vi "Main.vi"() -> ()   [LabVIEW 2014]
uses:
  SubVI/Configs/Temp/TempConfig.ctl
  SubVI/Configs/Count/Channel.ctl
  <vilib>/Utility/miscctls.llb/LVForegroundBackgroundColorsTypeDef.ctl
  SubVI/VBreakInitialCond.ctl
  SubVI/VBreakStopCondition.ctl
  <instrlib>/Agilent 532XX Series/Public/Configure/Measurement/Configure Measurement (Totalize Timed).vi
  <instrlib>/Agilent 532XX Series/Public/Configure/Configure Channel (Slop).vi
  <instrlib>/Agilent 532XX Series/Public/Configure/Configure Channel (Auto Threshold Voltage).vi
  <instrlib>/Agilent 532XX Series/Public/Data/Read Measurement (Statistics).vi
  <instrlib>/Agilent 532XX Series/Public/Configure/Measurement/Configure Measurement (Time Interval).vi
  <instrlib>/Agilent 532XX Series/Public/Data/Read Measurement (Multiple).vi
  <vilib>/Utility/file.llb/Write To Spreadsheet File (DBL).vi
  <instrlib>/Agilent 532XX Series/Agilent 532XX Series.lvlib
  <vilib>/Analysis/NI_AALPro.lvlib
panel:
  in  "Tab Control":enum32{"Manuel", "Auto", "Configs"}(tab)
  out "Temp":dbl
  in  "Ilim":dbl
  in  "Range":dbl
  in  "V":dbl
  in  "V On/Off":bool
  in  "Channel":i32(ring)=1 items=["Channel 1"=1, "Channel 2"=2]
  out "Vbreak":dbl
  out "Count":dbl
  in  "Count Max":dbl
  in  "Vmax":dbl
  in  "Count Min":dbl
  in  "Time Totalize":dbl
  in  "Level":dbl
  in  "VBreakStart":bool
  in  "Channel":i32(ring)=1 items=["Channel 1"=1, "Channel 2"=2]
  in  "Points":i32
  out "Histogramme":T1(graph)
  in  "Max":dbl
  in  "Min":dbl
  in  "Bean":i32
  in  "StartHistogramme":bool
  in  "Sauvegarde":path
  in  "StartStatCount":bool
  out "Max":dbl
  out "Min":dbl
  out "Ecart type":dbl
  out "Moyenne":dbl
  in  "Points":i32
  in  "Totalize Timed (s)":dbl
  in  "On / Off":bool
  in  "SetPoint":dbl
  in  "ConfigCounts":T3={"OK Button"=FALSE, "Channel1"={"AutoLevel"=FALSE, "Thresold"=1.0, "Active Edge"=1, "Impedance "=1000000.0, "Voltage Range"=5.0}, "Channel2"={"AutoLevel"=FALSE, "Thresold"=1.0, "Active Edge"=1, "Impedance "=1000000.0, "Voltage Range"=5.0}} {"Channel2"."Impedance" items=["50"=50.0, "1E+6"=1000000.0]; "Channel2"."Active Edge" items=["Positive", "Negative"]; "Channel1"."Impedance" items=["50"=50.0, "1E+6"=1000000.0]; "Channel1"."Active Edge" items=["Positive", "Negative"]}
  in  "Edit Temp Config":bool caption="Blank Button"
  in  "Combo Box":string(combo)
  out "TempConfig":T4
  in  "Stop Button":bool
  # "Tek Controler"
  # "Picoamp"
  # "Histogramme"
  # "Stat Count"
  # "Histograme"
  # "VBreak"
  # "Tec config"
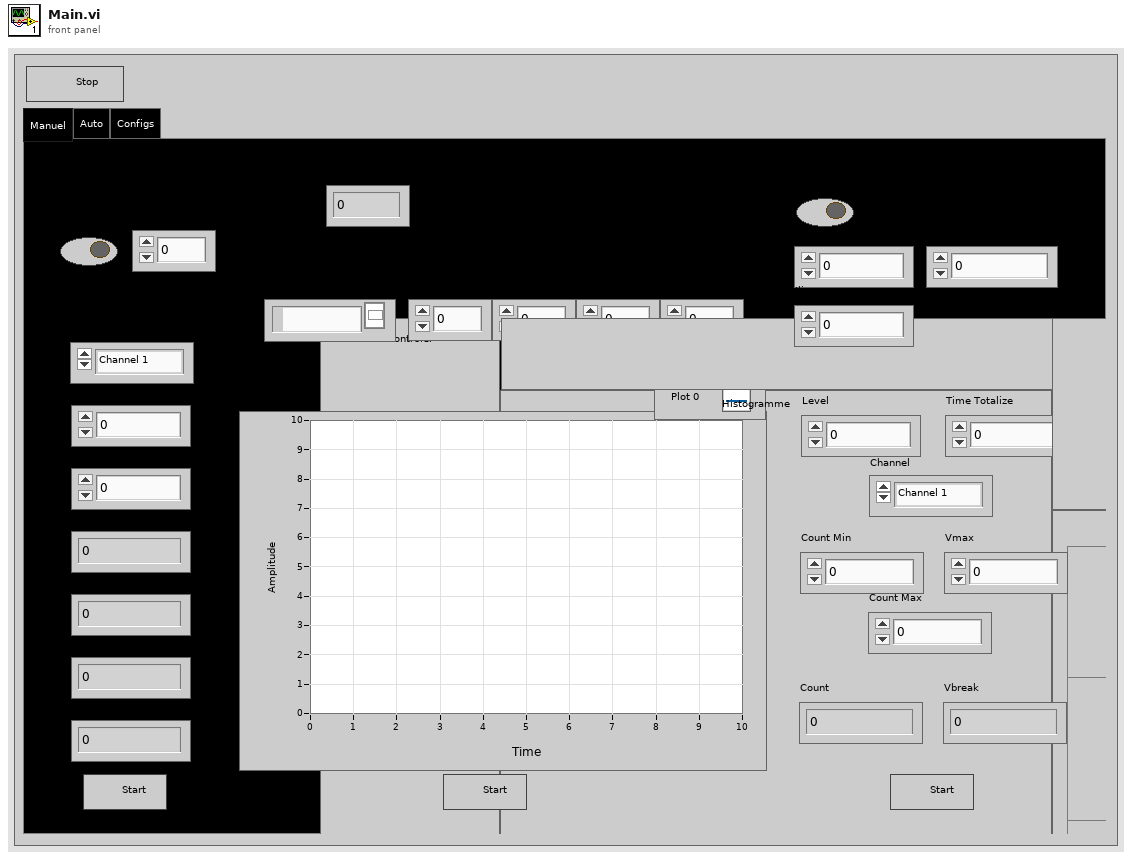
[diagram p1: front panel]
types:
  T1 = cluster{"X Values":dbl[], "Histogram: h(x)":i32[]}
  T2 = typedef "Channel.ctl" = cluster{"AutoLevel":bool, "Thresold":dbl, "Active Edge":i32, "Impedance ":dbl, "Voltage Range":dbl}
  T3 = cluster{"OK Button":bool, "Channel1":T2, "Channel2":T2}
  T4 = typedef "TempConfig.ctl" = cluster{"Name":string, "Thi":dbl, "Tlow":dbl, "Tstartup":dbl, "P":dbl, "I":dbl, "D":dbl, "Ilim":dbl, "Vlim":dbl, "Default":bool}
  T5 = typedef "LVForegroundBackgroundColorsTypeDef.ctl" = cluster{"Foreground Color":u32, "Background Color":u32}
  T6 = typedef "VBreakStopCondition.ctl" = cluster{"Count Min":dbl, "Count Max":dbl, "Vmax":dbl}
  T7 = typedef "VBreakInitialCond.ctl" = cluster{"Range":dbl, "Ilim":dbl, "Level":dbl, "Channel":i32, "Timed Totalize":dbl}
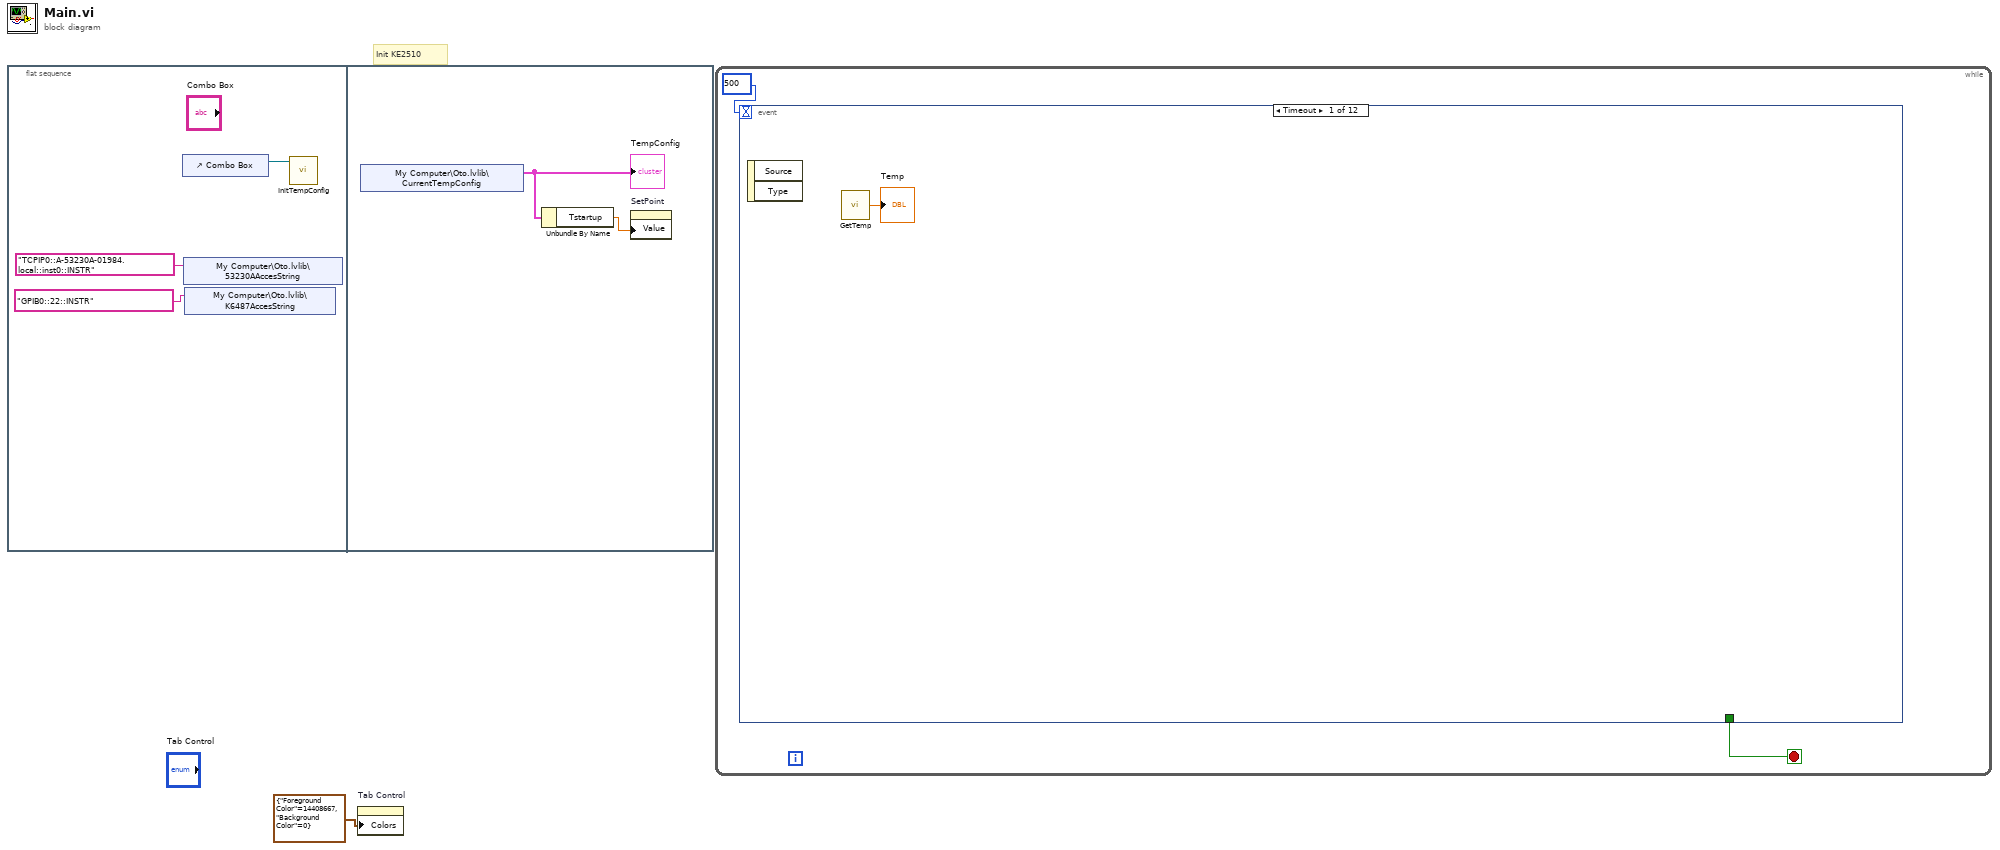
[diagram p0: block diagram]
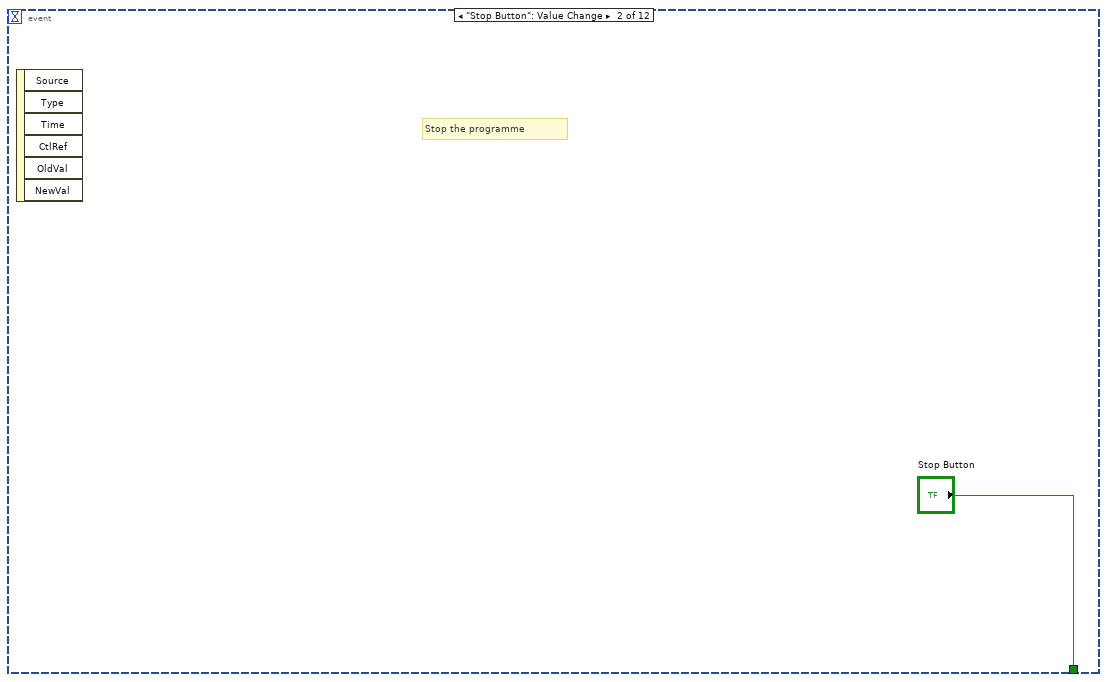
[diagram p2: hidden frame]
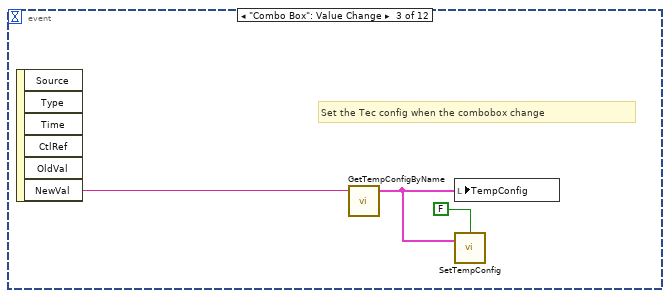
[diagram p3: hidden frame]
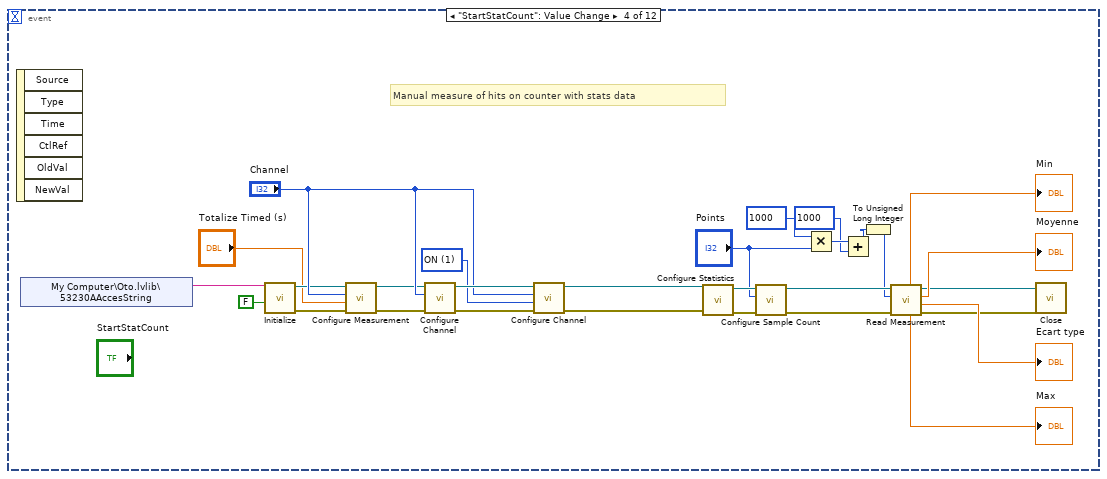
[diagram p4: hidden frame]
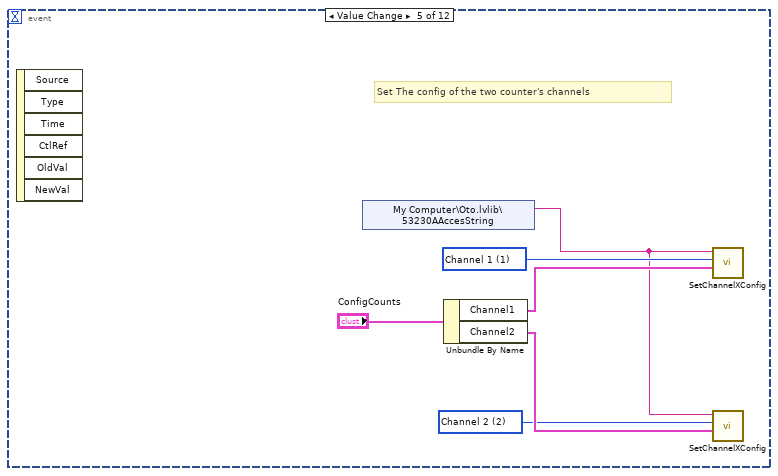
[diagram p5: hidden frame]
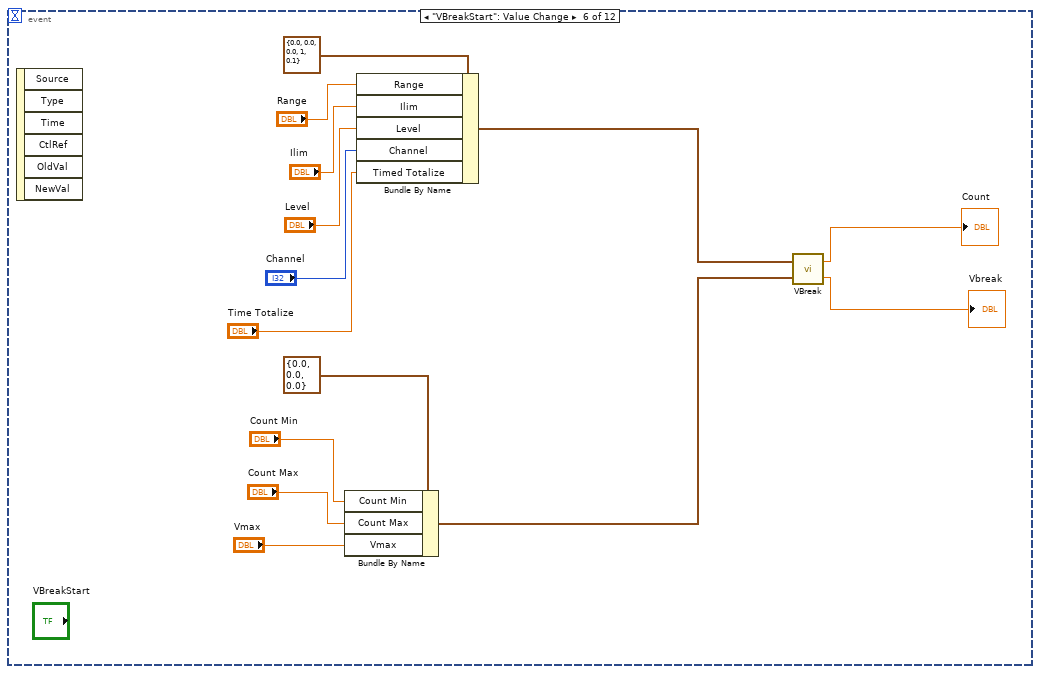
[diagram p6: hidden frame]
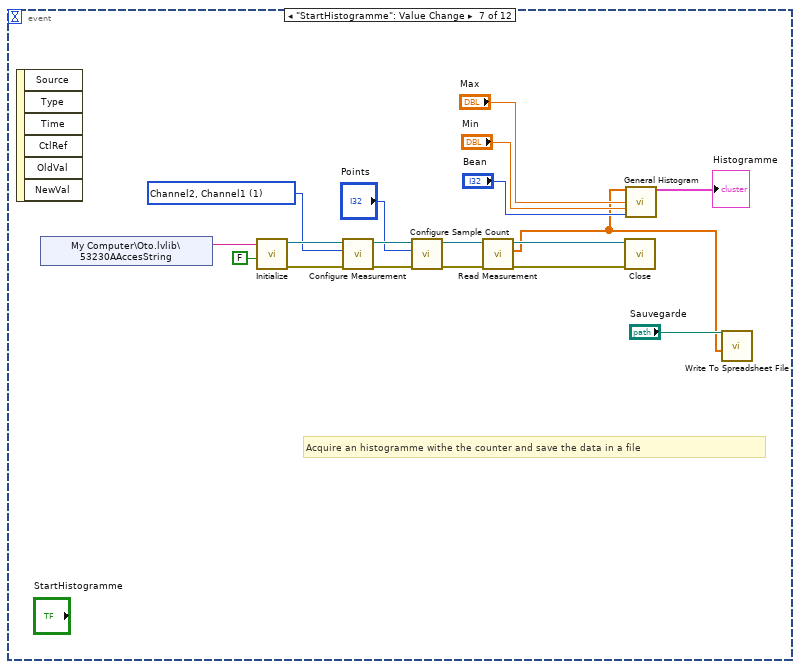
[diagram p7: hidden frame]
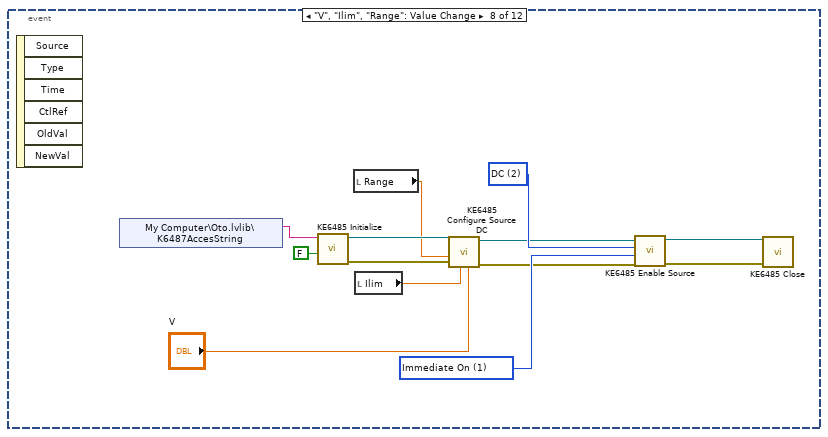
[diagram p8: hidden frame]
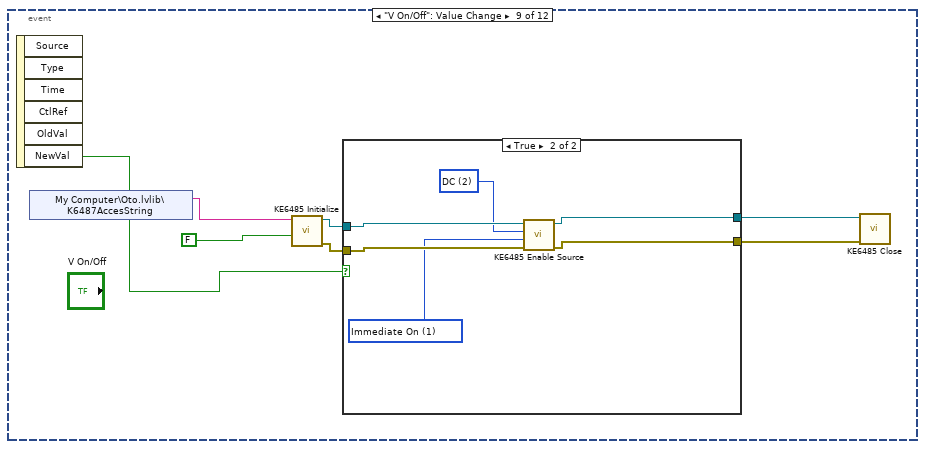
[diagram p9: hidden frame]
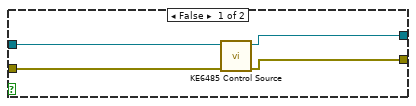
[diagram p10: hidden frame]
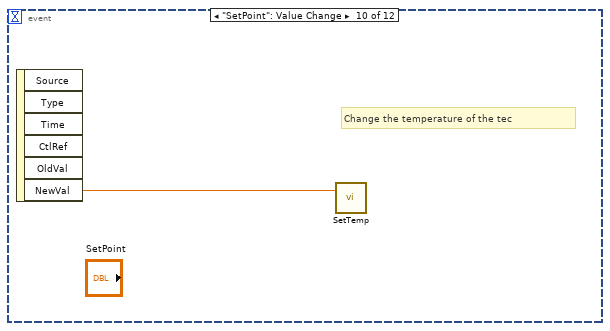
[diagram p11: hidden frame]
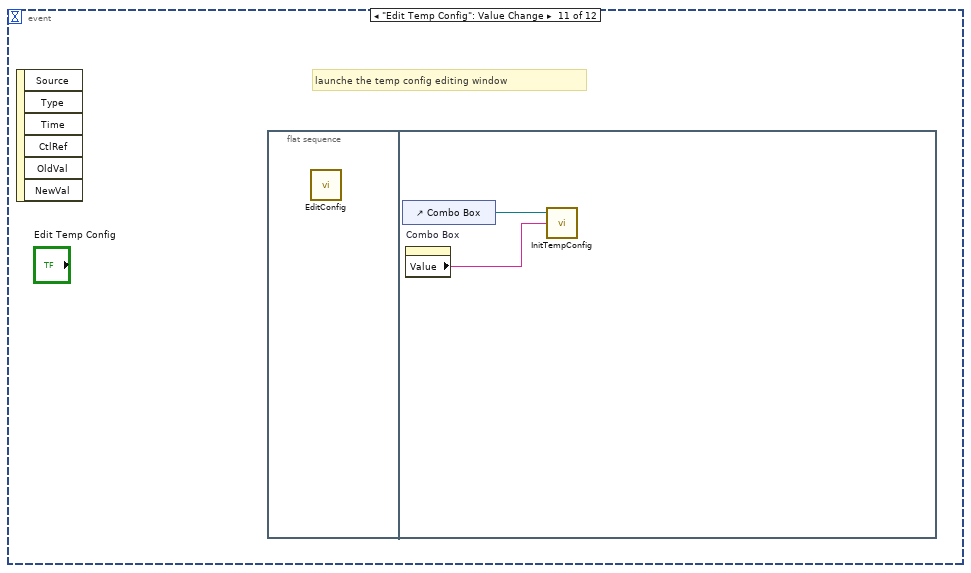
[diagram p12: hidden frame]
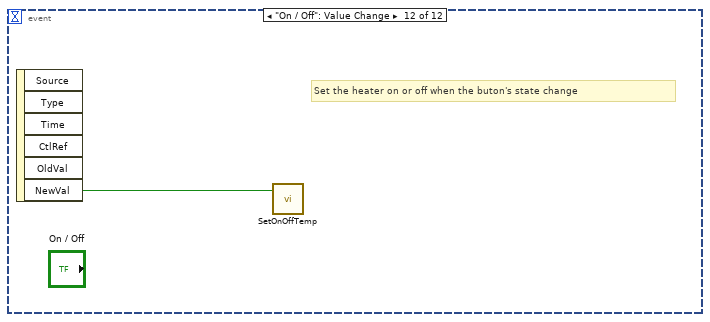
[diagram p13: hidden frame]
diagram:
  # "Init KE2510"
  n1 = flat-sequence {
    frame #0 {
      n2 = control-ref of="Combo Box"() -> (w4:refnum<vi>)
      n3 = shared-variable "My Computer\\Oto.lvlib\\53230AAccesString"("TCPIP0::A-53230A-01984.local::inst0::INSTR" ("K6487AccesString")) -> ()  [unwired: 1 in, 1 out]
      n4 = shared-variable "My Computer\\Oto.lvlib\\K6487AccesString"("GPIB0::22::INSTR" ("K6487AccesString")) -> ()  [unwired: 1 in, 1 out]
      n5 = call "InitTempConfig.vi"("CmbBox Refnum"=w4) -> ()  [unwired: 2 in, 1 out]
    }
    frame #1 {
      n6 = shared-variable "My Computer\\Oto.lvlib\\CurrentTempConfig"() -> (w5:T4)  [unwired: 1 in, 1 out]
      "TempConfig" <- w5
      n7 = Unbundle By Name(w5) -> ("Tstartup"=w6:dbl)
      n8 = property on="SetPoint" class="DigNum (strict)"("Value"=w6) -> ()  [unwired: 2 in, 2 out]
    }
  }
  n9 = property on="Tab Control" class="TabCtl (strict)"("Colors"=T5 {"Foreground Color"=14408667, "Background Color"=0}) -> ()  [unwired: 2 in, 2 out]
  n10 = while {
    stop <- w8 stop-if-true
    n11 = event shown="[0] Timeout" {
      selector: _ -> [_ _ _ _ _ _ _ _ _ _ _ _]
      dyn-events: _ -> [_ _ _ _ _ _ _ _ _ _ _ _]
      timeout: 500 -> [_ _ _ _ _ _ _ _ _ _ _ _]
      tunnel: [_ "Stop Button" _ _ _ _ _ _ _ _ _ _] -> w8
      event Timeout {
        n12 = event-data() -> ()  [unwired: 1 in, 2 out]
        n13 = call "GetTemp.vi"() -> ("result"=→"Temp":dbl)
      }
      event "Stop Button": Value Change {
        # "Stop the programme"
        n14 = event-data() -> ()  [unwired: 1 in, 6 out]
      }
      event "Combo Box": Value Change {
        # "Set the Tec config when the combobox change"
        n15 = event-data() -> ("NewVal"=w13:string)  [unwired: 1 in, 5 out]
        n16 = call "GetTempConfigByName.vi"("Name"=w13) -> ("TempConfig"=w12:T4)  [unwired: 2 in, 2 out]
        n17 = local write "TempConfig"(w12) -> ()
        n18 = call "SetTempConfig.vi"("Boolean"=FALSE, "Temp Configuration"=w12) -> ()  [unwired: 1 in, 1 out]
      }
      event "StartStatCount": Value Change {
        w22 = 1 items=["OFF", "ON", "ONCE"] ("Enable Auto-leveling (1: ON)")
        # "Manual measure of hits on counter with stats data"
        n19 = event-data() -> ()  [unwired: 1 in, 6 out]
        n20 = shared-variable "My Computer\\Oto.lvlib\\53230AAccesString"() -> (w42:string)  [unwired: 1 in, 1 out]
        n21 = call <instrlib>:"Initialize.vi"("Reset (True)"=FALSE, "VISA resource name"=w42) -> ("error out"=w19:errorcluster, "VISA resource name out"=w20:refnum<visa-resource-name>)  [unwired: 8 in]
        n22 = call-poly <instrlib>:"Configure Measurement.vi"("error in (no error)"=w19, "Timed Totalize (0.1 s)"="Totalize Timed (s)", "Channel (1: Channel 1)"="Channel", "VISA resource name"=w20) -> ("error out"=w17:errorcluster, "VISA resource name out"=w18:refnum<visa-resource-name>)  [unwired: 6 in]
        n23 = call-poly <instrlib>:"Configure Channel.vi"("error in (no error)"=w17, "Channel (1: Channel 1)"="Channel", "VISA resource name"=w18) -> ("error out"=w23:errorcluster, "VISA resource name out"=w24:refnum<visa-resource-name>)  [unwired: 7 in]
        n24 = call-poly <instrlib>:"Configure Channel.vi"("error in (no error)"=w23, "Enable Auto-leveling (1: ON)"=w22, "Channel (1: Channel 1)"="Channel", "VISA resource name"=w24) -> ("error out"=w14:errorcluster, "VISA resource name out"=w15:refnum<visa-resource-name>)  [unwired: 6 in]
        n25 = call <instrlib>:"Configure Statistics.vi"("error in (no error)"=w14, "VISA resource name"=w15) -> ("error out"=w40:errorcluster, "VISA resource name out"=w39:refnum<visa-resource-name>)  [unwired: 8 in]
        n26 = call <instrlib>:"Configure Sample Count.vi"("error in (no error)"=w40, "Sample Count (1)"="Points", "VISA resource name"=w39) -> ("error out"=w38:errorcluster, "VISA resource name out"=w37:refnum<visa-resource-name>)  [unwired: 7 in]
        n27 = Multiply(x=1000, y="Points") -> (x*y=w28:i32)
        n28 = Add(x=w28, y=1000) -> (x+y=w26:i32)
        n29 = To Unsigned Long Integer(number=w26) -> (unsigned 32bit integer=w25:u32)
        n30 = call-poly <instrlib>:"Read Measurement.vi"("error in (no error)"=w38, "Timeout (10000 ms)"=w25, "VISA resource name"=w37) -> ("error out"=w31:errorcluster, "Standard Deviation"=→"Ecart type":dbl, "Mean"=→"Moyenne":dbl, "VISA resource name out"=w32:refnum<visa-resource-name>, "Maximum"=→"Max":dbl, "Minimum"=→"Min":dbl)  [unwired: 3 in]
        n31 = call <instrlib>:"Close.vi"("error in (no error)"=w31, "VISA resource name"=w32) -> ()  [unwired: 9 in, 1 out]
      }
      event "ConfigCounts.OK Button": Value Change {
        w43 = 2 items=["Channel 1"=1, "Channel 2"=2] ("Channel (1: Channel 1)")
        w45 = 1 items=["Channel 1"=1, "Channel 2"=2] ("Channel (1: Channel 1)")
        # "Set The config of the two counter's channels"
        n32 = event-data() -> ()  [unwired: 1 in, 6 out]
        n33 = shared-variable "My Computer\\Oto.lvlib\\53230AAccesString"() -> (w44:string)  [unwired: 1 in, 1 out]
        n34 = Unbundle By Name("ConfigCounts") -> ("Channel1"=w47:T2, "Channel2"=w46:T2)
        n35 = call "SetChannelXConfig.vi"("Channel1"=w47, "Channel (1: Channel 1)"=w45, "VISA Ressource"=w44) -> ()  [unwired: 1 in, 1 out]
        n36 = call "SetChannelXConfig.vi"("Channel1"=w46, "Channel (1: Channel 1)"=w43, "VISA Ressource"=w44) -> ()  [unwired: 1 in, 1 out]
      }
      event "VBreakStart": Value Change {
        n37 = event-data() -> ()  [unwired: 1 in, 6 out]
        n38 = Bundle By Name(cluster=T6 {"Count Min"=0.0, "Count Max"=0.0, "Vmax"=0.0} ("Condition d'arret"), "Count Min"="Count Min", "Count Max"="Count Max", "Vmax"="Vmax") -> (w49:T6)
        n39 = Bundle By Name(cluster=T7 {"Range"=0.0, "Ilim"=0.0, "Level"=0.0, "Channel"=1, "Timed Totalize"=0.1} ("Condition Initial"), "Range"="Range", "Ilim"="Ilim", "Level"="Level", "Channel"="Channel", "Timed Totalize"="Time Totalize") -> (w54:T7)
        n40 = call "VBreak.vi"("Condition d'arret"=w49, "Condition Initial"=w54) -> ("VBreak"=→"Vbreak":dbl, "Count"=→"Count":dbl)
      }
      event "StartHistogramme": Value Change {
        w76 = 1 items=["Channel1, Channel2", "Channel2, Channel1", " Channel1", "Channel2"] ("Measurement Channels (0: Channel1, Channel2)")
        # "Acquire an histogramme withe the counter and save the data in a file"
        n41 = event-data() -> ()  [unwired: 1 in, 6 out]
        n42 = shared-variable "My Computer\\Oto.lvlib\\53230AAccesString"() -> (w80:string)  [unwired: 1 in, 1 out]
        n43 = call <instrlib>:"Initialize.vi"("Reset (True)"=FALSE, "VISA resource name"=w80) -> ("error out"=w78:errorcluster, "VISA resource name out"=w77:refnum<visa-resource-name>)  [unwired: 8 in]
        n44 = call-poly <instrlib>:"Configure Measurement.vi"("error in (no error)"=w78, "Measurement Channels (0: Channel1, Channel2)"=w76, "VISA resource name"=w77) -> ("error out"=w75:errorcluster, "VISA resource name out"=w74:refnum<visa-resource-name>)  [unwired: 7 in]
        n45 = call <instrlib>:"Configure Sample Count.vi"("error in (no error)"=w75, "Sample Count (1)"="Points", "VISA resource name"=w74) -> ("error out"=w72:errorcluster, "VISA resource name out"=w71:refnum<visa-resource-name>)  [unwired: 7 in]
        n46 = call-poly <instrlib>:"Read Measurement.vi"("error in (no error)"=w72, "VISA resource name"=w71) -> ("error out"=w70:errorcluster, "Measurements"=w63:dbl[], "VISA resource name out"=w69:refnum<visa-resource-name>)  [unwired: 7 in]
        n47 = call <instrlib>:"Close.vi"("error in (no error)"=w70, "VISA resource name"=w69) -> ()  [unwired: 9 in, 1 out]
        n48 = call <vilib>:"General Histogram.vi"("X"=w63, "max"="Max", "min"="Min", "# bins"="Bean") -> ("Histogram Graph"=→"Histogramme":T1)  [unwired: 7 in, 4 out]
        n49 = call-poly <vilib>:"Write To Spreadsheet File.vi"("1D data"=w63, "file path (dialog if empty)"="Sauvegarde") -> ()  [unwired: 6 in, 1 out]
      }
      event "V", "Ilim", "Range": Value Change {
        w85 = 1 items=["Immediate On"=1, "Immediate Off"=2, "Immediate Standby"=4, "Auto Sync Enabled"=65536, "Auto Sync Disabled"=131072] ("output action")
        w86 = 2 items=["Bias"=1, "DC"=2, "Ramp"=4] ("generator")
        n50 = event-data() -> ()  [unwired: 1 in, 6 out]
        n51 = shared-variable "My Computer\\Oto.lvlib\\K6487AccesString"() -> (w91:string)  [unwired: 1 in, 1 out]
        n52 = call <instrlib>:"KE6485 Initialize.vi"("reset device"=FALSE, "resource name"=w91) -> ("error out"=w92:errorcluster, "instrument handle out"=w93:refnum<k15>)  [unwired: 8 in]
        n53 = local read "Range"() -> (w88:dbl)
        n54 = local read "Ilim"() -> (w87:dbl)
        n55 = call <instrlib>:"KE6485 Configure Source DC.vi"("level"="V", "compliance limit"=w87, "error in (no error)"=w92, "range"=w88, "instrument handle"=w93) -> ("error out"=w84:errorcluster, "instrument handle out"=w83:refnum<k15>)  [unwired: 5 in]
        n56 = call <instrlib>:"KE6485 Enable Source.vi"("error in (no error)"=w84, "output action"=w85, "generator"=w86, "instrument handle"=w83) -> ("error out"=w81:errorcluster, "instrument handle out"=w82:refnum<k15>)  [unwired: 6 in]
        n57 = call <instrlib>:"KE6485 Close.vi"("error in (no error)"=w81, "instrument handle"=w82) -> ()  [unwired: 9 in, 1 out]
      }
      event "V On/Off": Value Change {
        n58 = event-data() -> ("NewVal"=w98:bool)  [unwired: 1 in, 5 out]
        n59 = shared-variable "My Computer\\Oto.lvlib\\K6487AccesString"() -> (w99:string)  [unwired: 1 in, 1 out]
        n60 = call <instrlib>:"KE6485 Initialize.vi"("reset device"=FALSE, "resource name"=w99) -> ("error out"=w96:errorcluster, "instrument handle out"=w97:refnum<k15>)  [unwired: 8 in]
        n61 = case shown="True" w98 {
          tunnel: w97 -> [w104 w110]
          tunnel: w96 -> [w103 w109]
          tunnel: [w102 w106] -> w95
          tunnel: [w101 w105] -> w94
          frame False {
            n62 = call <instrlib>:"KE6485 Control Source.vi"("error in (no error)"=w103, "instrument handle"=w104) -> ("error out"=w101:errorcluster, "instrument handle out"=w102:refnum<k15>)  [unwired: 8 in]
          }
          frame True {
            w107 = 2 items=["Bias"=1, "DC"=2, "Ramp"=4] ("generator")
            w108 = 1 items=["Immediate On"=1, "Immediate Off"=2, "Immediate Standby"=4, "Auto Sync Enabled"=65536, "Auto Sync Disabled"=131072] ("output action")
            n63 = call <instrlib>:"KE6485 Enable Source.vi"("error in (no error)"=w109, "output action"=w108, "generator"=w107, "instrument handle"=w110) -> ("error out"=w105:errorcluster, "instrument handle out"=w106:refnum<k15>)  [unwired: 6 in]
          }
        }
        n64 = call <instrlib>:"KE6485 Close.vi"("error in (no error)"=w94, "instrument handle"=w95) -> ()  [unwired: 9 in, 1 out]
      }
      event "SetPoint": Value Change {
        # "Change the temperature of the tec"
        n65 = event-data() -> ("NewVal"=w111:dbl)  [unwired: 1 in, 5 out]
        n66 = call "SetTemp.vi"("Numeric Control"=w111) -> ()  [unwired: 1 in, 1 out]
      }
      event "Edit Temp Config": Value Change {
        # "launche the temp config editing window"
        n67 = event-data() -> ()  [unwired: 1 in, 6 out]
        n68 = flat-sequence {
          frame #0 {
            n69 = call "EditConfig.vi"() -> ()  [unwired: 12 in]
          }
          frame #1 {
            n70 = control-ref of="Combo Box"() -> (w113:refnum<vi>)
            n71 = property on="Combo Box" class="CmbBox"() -> ("Value"=w112:string)  [unwired: 2 in, 2 out]
            n72 = call "InitTempConfig.vi"("ConfigName"=w112, "CmbBox Refnum"=w113) -> ()  [unwired: 1 in, 1 out]
          }
        }
      }
      event "On / Off": Value Change {
        # "Set the heater on or off when the buton's state change"
        n73 = event-data() -> ("NewVal"=w114:bool)  [unwired: 1 in, 5 out]
        n74 = call "SetOnOffTemp.vi"("Boolean"=w114) -> ()  [unwired: 1 in, 1 out]
      }
    }
  }
